vi "GetInitialDataTC110.vi"(8 "error in (no error)":errorcluster, 9 "Map":map{T1, variant}(c390), 10 "Adress of unit":u16, 11 "VISA Refnum in":refnum<visa-resource-name>) -> (0 "error out":errorcluster, 2 "data map":map{T1, variant}(c390), 3 "VISA session out":refnum<visa-resource-name>)   [LabVIEW 2019]
uses:
  PfeifferTC110Cmds.ctl
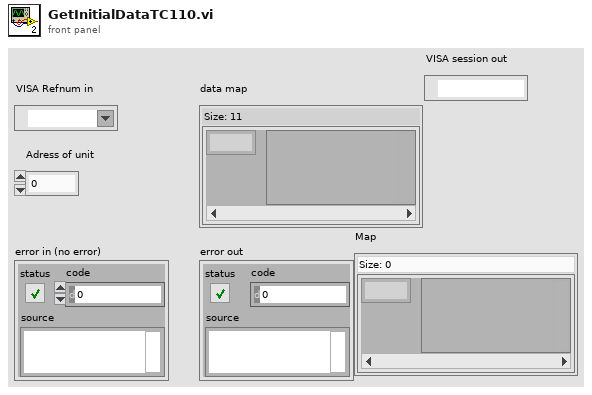
[diagram p1: front panel]
types:
  T1 = typedef "PfeifferTC110Cmds.ctl" = enum16{"Standby", "AckError", "Run", "Motor", "SpdSwPtAtt", "ErrorCode", "OvTempElec", "OvTempPump", "SetSpdAtt", "PumpAccel", "ActualSpdHz", "DrvCurrent", "OpHrsPump", "FwVersion", "DrvVoltage", "OpHrsElec", "NominalSpd", "DrvPower", "PumpCycles", "TempElec", "TempPmpBot", "AccelDecel", "TempBearing", "TempMotor", "ElecName", "HWVersion", "SetRotSpdRPM", "ActualSpdRPM", "NominalSpdRPM"}
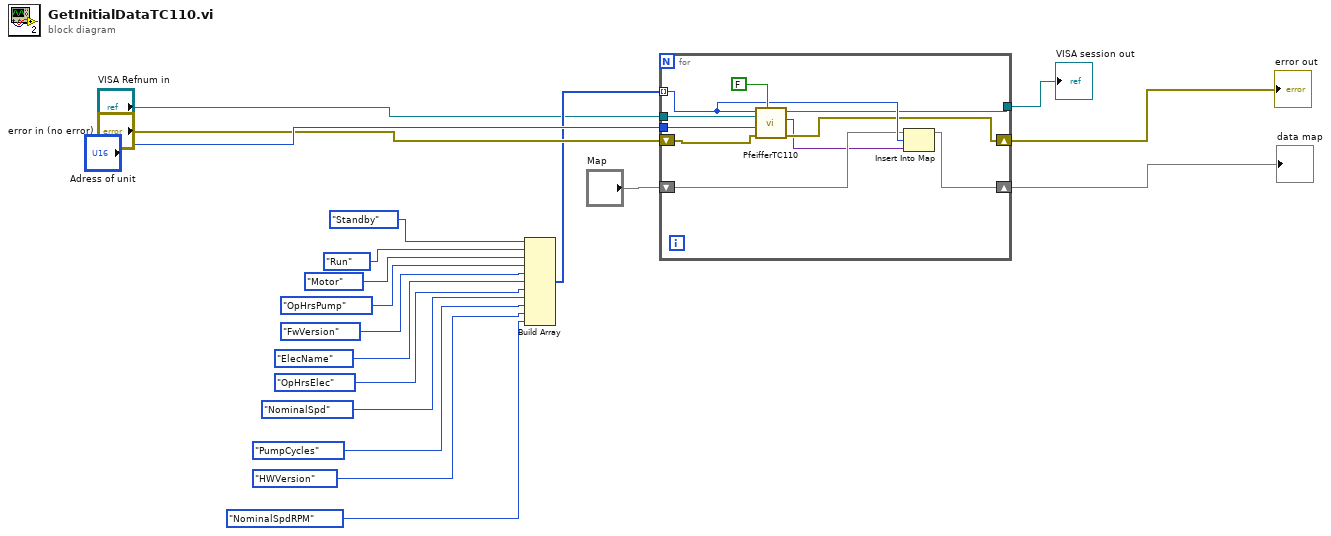
[diagram p0: block diagram]
diagram:
  n1 = Build Array(PfeifferTC110Cmds."Standby" ("CMD ID"), PfeifferTC110Cmds."Run" ("CMD ID"), PfeifferTC110Cmds."Motor" ("CMD ID"), PfeifferTC110Cmds."OpHrsPump" ("CMD ID"), PfeifferTC110Cmds."FwVersion" ("CMD ID"), PfeifferTC110Cmds."ElecName" ("CMD ID"), PfeifferTC110Cmds."OpHrsElec" ("CMD ID"), PfeifferTC110Cmds."NominalSpd" ("CMD ID"), PfeifferTC110Cmds."PumpCycles" ("CMD ID"), PfeifferTC110Cmds."HWVersion" ("CMD ID"), PfeifferTC110Cmds."NominalSpdRPM" ("CMD ID")) -> (w14:T1[])
  n2 = for {
    tunnel: "VISA Refnum in" -> [w29]
    tunnel: w14 -> [w25] mode=indexing
    shift-right: [w22] -> w19
    shift-left: "error in (no error)" -> [w28]
    tunnel: "Adress of unit" -> [w26]
    shift-right: [w23] -> w18
    shift-left: "Map" -> [w24]
    tunnel: [w20] -> w2
    n3 = call "PfeifferTC110.vi"("Write?"=FALSE, "error in"=w28, "Adress"=w26, "VISA session"=w29, "CMD ID"=w25) -> ("error out"=w22:errorcluster, "Response"=w21:variant, "VISA session out"=w20:refnum<visa-resource-name>)  [unwired: 4 in]
    n4 = Insert Into Map(map in=w24, key=w25, value=w21) -> (map out=w23:map{T1, variant})  [unwired: 2 out]
  }
  "error out" <- w19
  "data map" <- w18
  "VISA session out" <- w2
